vi "channel Offset UI.vi"(11 "eventData":T1) -> (1 "offsets":dbl[](array[numeric]), 3 "changed?":bool)   [LabVIEW 2018]
uses:
  type defs/event data.ctl
  offsetTypes.ctl
  ICL-LabVIEW_General/data channels/parent class/channel type.ctl
  ICL-LabVIEW_General/data channels/data channels.lvlib
  ICL-LabVIEW_General/data channels/parent class/Data Channel.lvclass
panel:
  in  "Offset to value:":dbl
  in  "Channel to match:":u16(ring) items=["time", "gearbox", "Recirculation temp", "volute exit surface", "oil tank", "Inlet average", "Outlet average", "V-cone", "inlet pressure", "outlet pressure", "Motor speed", "V-cone DP", "Motor power", "Accelerometer", "Hotwire", "oil pressure", "butterfly valve position", "ball valve position", "Legacy speed", "new Vcone", "V-Cone: CR001", "pressure ratio", "Ambient pressure", "Ambient temperature"]
  in  "Offset type:":T2(ring)
  in  "create":bool
  in  "done":bool
  in  "cancel":bool
  in  "channelControl":T3(array[cluster])
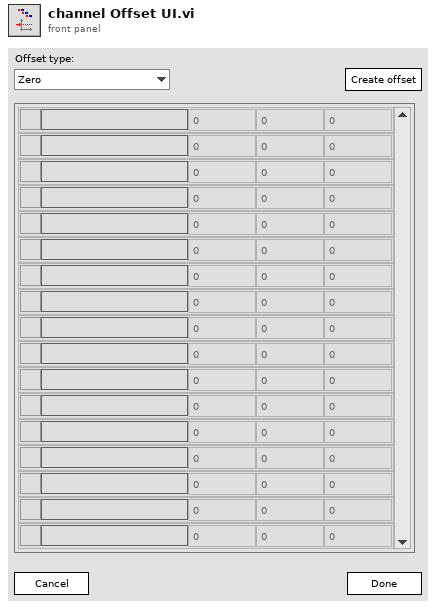
[diagram p1: front panel]
types:
  T1 = typedef "event data.ctl" = cluster{"menuRef":refnum<k9>, "channelConfigPath":path, "tempOffsets":dbl[]}
  T2 = enum16{"Zero", "Offset to value", "Offset to match channel", "Remove offset"}
  T3 = cluster{"select":bool, "channel":string, "value":dbl, "offset":dbl, "new value":dbl}[]
  T4 = typedef "data channels.lvlib/Data Channel.lvclass/channel type.ctl" = enum16{"acquisition", "output", "other"}
  T5 = typedef "offsetTypes.ctl" = enum16{"wait", "init", "createOffset", "done", "cancel"}
  T6 = cluster{"select":bool, "channel":string, "value":dbl, "offset":dbl, "offsetValue":dbl}
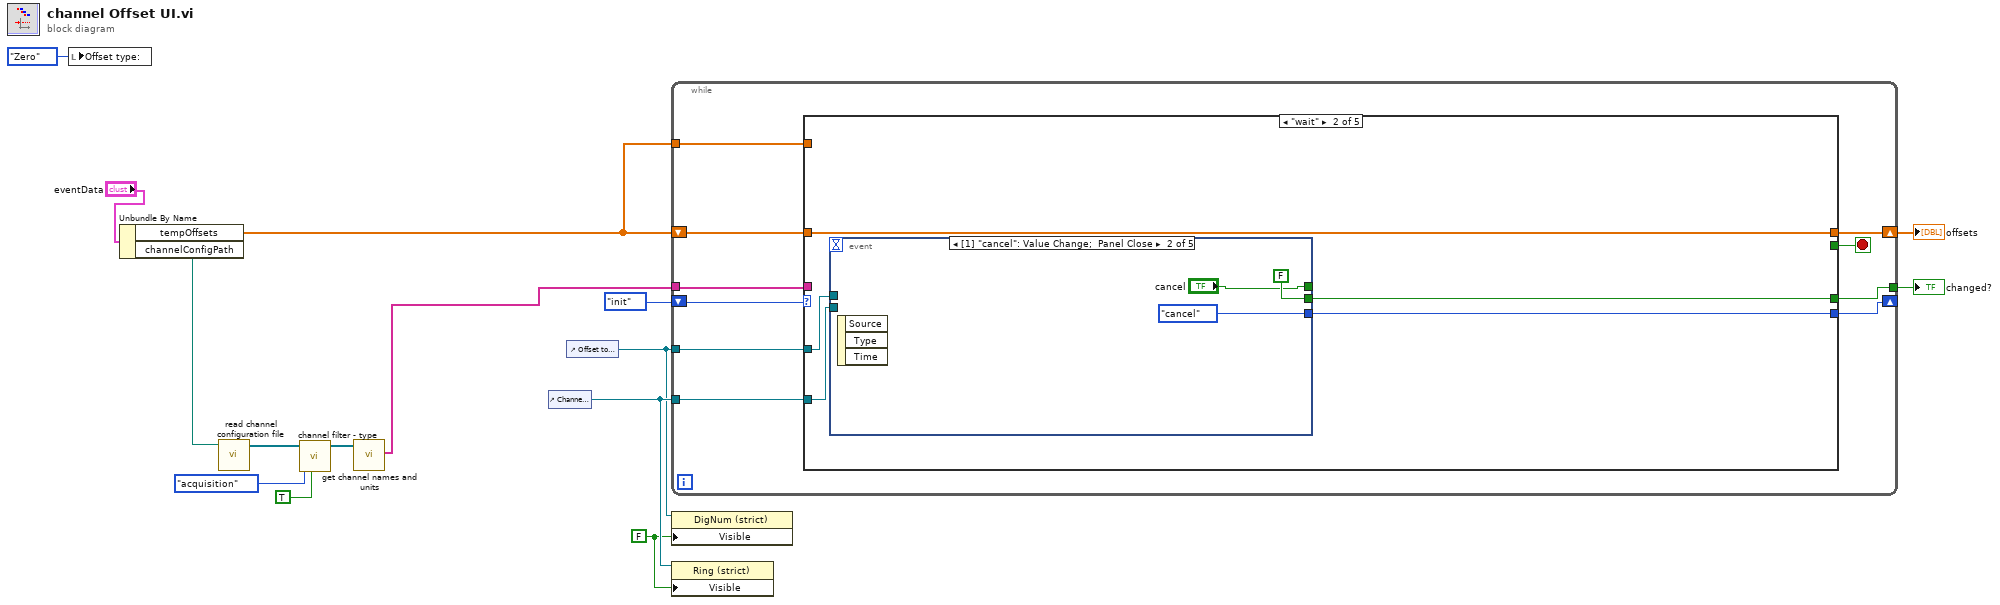
[diagram p0: block diagram]
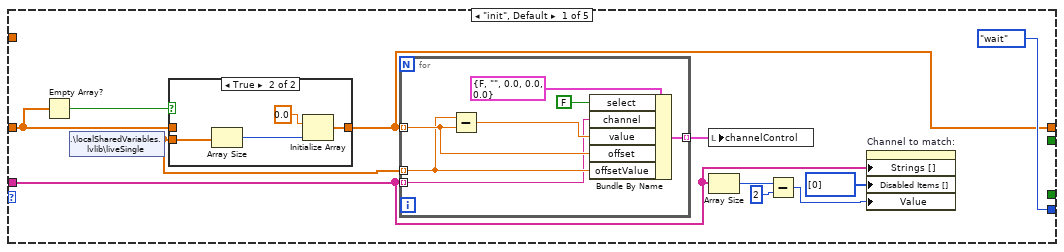
[diagram p2: hidden frame]
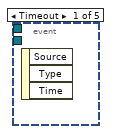
[diagram p4: hidden frame]
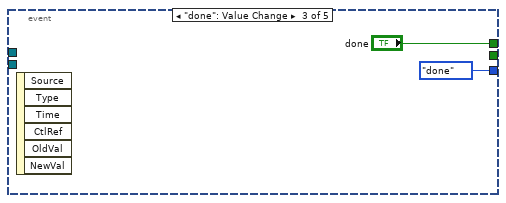
[diagram p5: hidden frame]
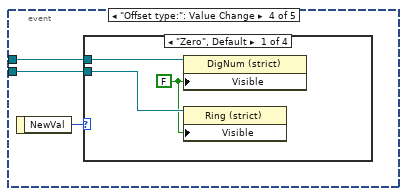
[diagram p6: hidden frame]
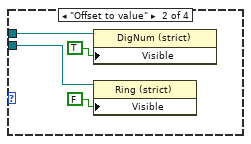
[diagram p7: hidden frame]
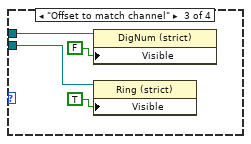
[diagram p8: hidden frame]
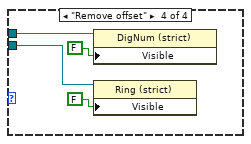
[diagram p9: hidden frame]
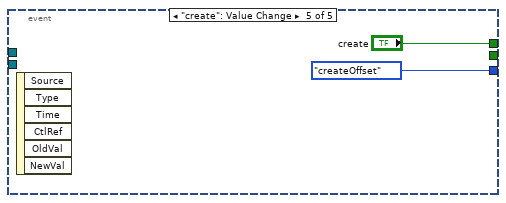
[diagram p10: hidden frame]
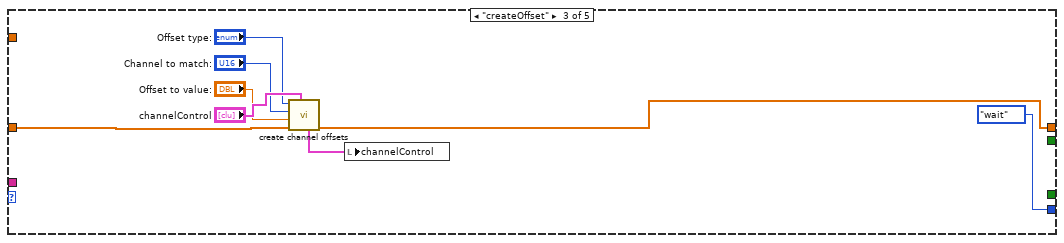
[diagram p11: hidden frame]
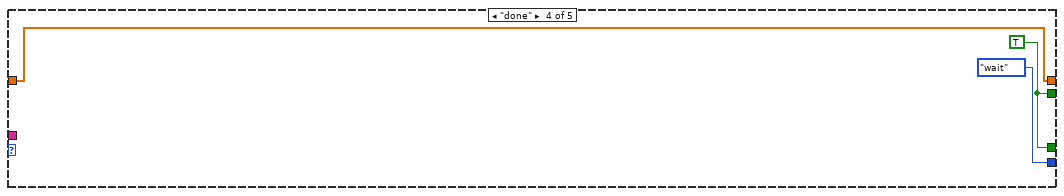
[diagram p12: hidden frame]
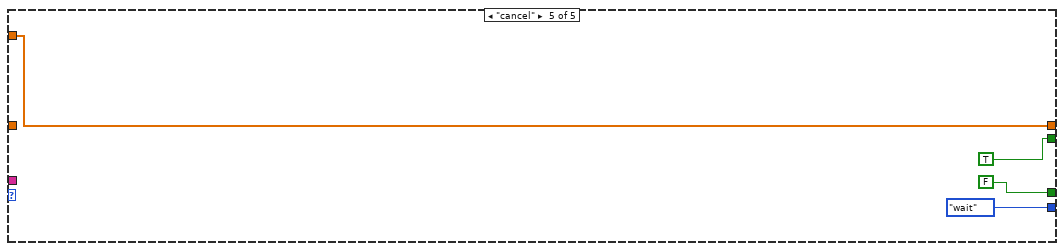
[diagram p13: hidden frame]
diagram:
  w12 = FALSE ("Visible")
  n1 = local write "Offset type:"(T2."Zero" ("Offset type:")) -> ()
  n2 = Unbundle By Name("eventData") -> ("tempOffsets"=w8:dbl[], "channelConfigPath"=w7:path)
  n3 = call "read channel configuration file.vi"("config file"=w7) -> ("channelsArray"=w6:refnum<class "Data Channel.lvclass">[])  [unwired: 8 in, 2 out]
  n4 = call "channel filter - type.vi"("activeOnly (F)"=TRUE, "channelType"=channel_type."acquisition", "channels"=w6) -> ("filteredChannels"=w4:refnum<class "Data Channel.lvclass">[])  [unwired: 6 in, 2 out]
  n5 = call "get channel names and units.vi"("channels"=w4) -> ("channelName"=w3:string[])  [unwired: 7 in, 3 out]
  n6 = control-ref of="Channel to match:"() -> (w14:refnum<vi>)
  n7 = control-ref of="Offset to value:"() -> (w13:refnum<vi>)
  n8 = while {
    shift-right: [w24] -> _
    shift-left: offsetTypes."init" -> [w25]
    tunnel: [w22] -> w10
    shift-right: [w21] -> w9
    shift-left: w8 -> [w20]
    tunnel: w14 -> [w19]
    tunnel: w13 -> [w18]
    tunnel: w3 -> [w17]
    tunnel: w8 -> [w16]
    stop <- w23 stop-if-true
    n9 = case shown="\"wait\"" w25 {
      tunnel: [offsetTypes."wait" w51 offsetTypes."wait" offsetTypes."wait" offsetTypes."wait"] -> w24
      tunnel: [_ _ _ w88 TRUE ("cancel")] -> w23
      tunnel: [_ w53 _ w88 FALSE ("cancel")] -> w22
      tunnel: [w29 w52 w84 w89 w90] -> w21
      tunnel: w20 -> [w28 w52 w85 w89 _]
      tunnel: w19 -> [_ w50 _ _ _]
      tunnel: w18 -> [_ w49 _ _ _]
      tunnel: w17 -> [w26 _ _ _ _]
      tunnel: w16 -> [_ _ _ _ w90]
      frame "init", Default {
        n10 = Empty Array?(array=w28) -> (empty?=w31:bool)
        n11 = shared-variable ".\\localSharedVariables.lvlib\\liveSingle"() -> (w30:dbl[])  [unwired: 1 in, 1 out]
        n12 = case shown="True" w31 {
          tunnel: w28 -> [w37 _]
          tunnel: w30 -> [_ w41]
          tunnel: [w37 w38] -> w29
          frame False {
          }
          frame True {
            n13 = Array Size(array=w41) -> (size(s)=w40:i32)
            n14 = Initialize Array(0.0 ("element"), w40) -> (w38:dbl[])
          }
        }
        n15 = for {
          tunnel: [w48] -> w36 mode=indexing
          tunnel: w30 -> [w44] mode=indexing
          tunnel: w29 -> [w45] mode=indexing
          tunnel: w26 -> [w42] mode=indexing
          n16 = Subtract(x=w44, y=w45) -> (x-y=w46:dbl)
          n17 = Bundle By Name(cluster=T6 {"select"=FALSE, "channel"="", "value"=0.0, "offset"=0.0, "offsetValue"=0.0} ("channelControl"), "select"=FALSE, "channel"=w42, "value"=w46, "offset"=w45, "offsetValue"=w44) -> (w48:T6)
        }
        n18 = local write "channelControl"(w36) -> ()
        n19 = Array Size(array=w26) -> (size(s)=w33:i32)
        n20 = Subtract(x=w33, y=2) -> (x-y=w27:i32)
        n21 = property on="Channel to match:" class="Ring (strict)"("Strings []"=w26, "Disabled Items []"=i32[] [0], "Value"=w27) -> ()  [unwired: 2 in, 2 out]
      }
      frame "wait" {
        n22 = event shown="[1] \"cancel\": Value Change;  Panel Close" {
          selector: _ -> [_ _ _ _ _]
          dyn-events: _ -> [_ _ _ _ _]
          timeout: _ -> [_ _ _ _ _]
          tunnel: [_ FALSE ("cancel") _ _ _] -> w53
          tunnel: [_ "cancel" "done" _ "create"] -> _
          tunnel: [_ offsetTypes."cancel" offsetTypes."done" _ offsetTypes."createOffset"] -> w51
          tunnel: w50 -> [_ _ _ w61 _]
          tunnel: w49 -> [_ _ _ w60 _]
          event Timeout {
            n23 = event-data() -> ()  [unwired: 1 in, 3 out]
          }
          event "cancel": Value Change; Panel Close {
            n24 = event-data() -> ()  [unwired: 1 in, 3 out]
          }
          event "done": Value Change {
            n25 = event-data() -> ()  [unwired: 1 in, 6 out]
          }
          event "Offset type:": Value Change {
            n26 = event-data() -> ("NewVal"=w59:T2)  [unwired: 1 in]
            n27 = case shown="\"Zero\", Default" w59 {
              tunnel: w61 -> [w64 w68 w72 w76]
              tunnel: w60 -> [w63 w67 w71 w75]
              frame "Zero", Default {
                w62 = FALSE ("Visible")
                n28 = property class="DigNum (strict)"(reference=w63, "Visible"=w62) -> ()  [unwired: 1 in, 2 out]
                n29 = property class="Ring (strict)"(reference=w64, "Visible"=w62) -> ()  [unwired: 1 in, 2 out]
              }
              frame "Offset to value" {
                n30 = property class="DigNum (strict)"(reference=w67, "Visible"=TRUE) -> ()  [unwired: 1 in, 2 out]
                n31 = property class="Ring (strict)"(reference=w68, "Visible"=FALSE) -> ()  [unwired: 1 in, 2 out]
              }
              frame "Offset to match channel" {
                n32 = property class="DigNum (strict)"(reference=w71, "Visible"=FALSE) -> ()  [unwired: 1 in, 2 out]
                n33 = property class="Ring (strict)"(reference=w72, "Visible"=TRUE) -> ()  [unwired: 1 in, 2 out]
              }
              frame "Remove offset" {
                n34 = property class="DigNum (strict)"(reference=w75, "Visible"=FALSE) -> ()  [unwired: 1 in, 2 out]
                n35 = property class="Ring (strict)"(reference=w76, "Visible"=FALSE) -> ()  [unwired: 1 in, 2 out]
              }
            }
          }
          event "create": Value Change {
            n36 = event-data() -> ()  [unwired: 1 in, 6 out]
          }
        }
      }
      frame "createOffset" {
        n37 = call "create channel offsets.vi"("channelControl"="channelControl", "offsets in"=w85, "Offset to value:"="Offset to value:", "Channel to match:"="Channel to match:", "Offset type:"="Offset type:") -> ("offsets out"=w84:dbl[], "updatedChannels"=w79:T3)  [unwired: 5 in]
        n38 = local write "channelControl"(w79) -> ()
      }
      frame "done" {
        w88 = TRUE ("cancel")
      }
      frame "cancel" {
      }
    }
  }
  "changed?" <- w10
  "offsets" <- w9
  n39 = property class="DigNum (strict)"(reference=w13, "Visible"=w12) -> ()  [unwired: 1 in, 2 out]
  n40 = property class="Ring (strict)"(reference=w14, "Visible"=w12) -> ()  [unwired: 1 in, 2 out]
